vi "tasklist_wait.vi"(8 "error in (no error)":errorcluster, 11 "pid":i32) -> (0 "error out":errorcluster)   [LabVIEW 2015, in "lv-bin-windows.lvlib" / "v1.lvlib"]
uses:
  v1.lvlib
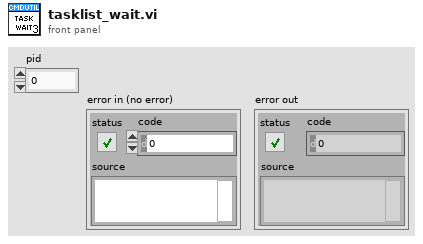
[diagram p1: front panel]
types:
  T1 = cluster{"image_name []":string[], "pid []":i32[], "session_name []":string[], "session_number []":i32[], "memory_usage []":dbl[]}
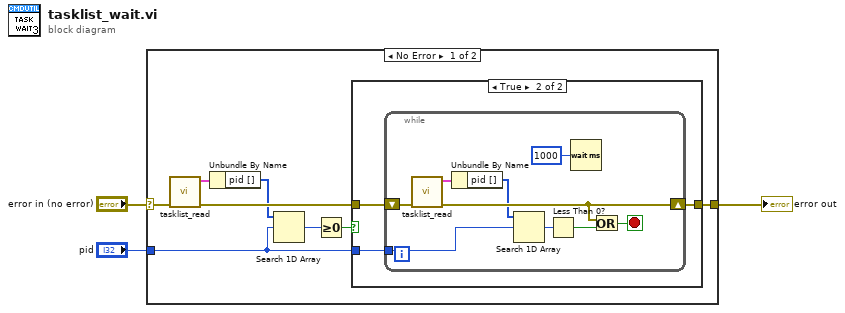
[diagram p0: block diagram]
diagram:
  n1 = case shown="No Error" "error in (no error)" {
    selector: "error in (no error)" -> [w6 w25]
    tunnel: "pid" -> [w7 _]
    tunnel: [w5 w25] -> w1
    frame No Error {
      n2 = call "tasklist_read.vi"("error in (no error)"=w6) -> ("error out"=w11:errorcluster, "tasklist"=w10:T1)  [unwired: 9 in]
      n3 = Unbundle By Name(w10) -> ("pid []"=w9:i32[])
      n4 = Search 1D Array(1D array=w9, element=w7) -> (index of element=w8:i32)  [unwired: 1 in]
      n5 = Greater Or Equal To 0?(x=w8) -> (x >= 0?=w4:bool)
      n6 = case shown="True" w4 {
        tunnel: w11 -> [w12 w15]
        tunnel: w7 -> [_ w14]
        tunnel: [w12 w13] -> w5
        frame False {
        }
        frame True {
          n7 = while {
            tunnel: w14 -> [w16]
            shift-right: [w24] -> w13
            shift-left: w15 -> [w17]
            stop <- w18 stop-if-true
            n8 = call "tasklist_read.vi"("error in (no error)"=w17) -> ("error out"=w24:errorcluster, "tasklist"=w21:T1)  [unwired: 9 in]
            n9 = Unbundle By Name(w21) -> ("pid []"=w22:i32[])
            n10 = Search 1D Array(1D array=w22, element=w16) -> (index of element=w23:i32)  [unwired: 1 in]
            n11 = Less Than 0?(x=w23) -> (x < 0?=w19:bool)
            n12 = Wait (ms)(milliseconds to wait=u32 1000) -> ()  [unwired: 1 out]
            n13 = Or(x=w24, y=w19) -> (x .or. y?=w18:bool)
          }
        }
      }
    }
    frame Error {
    }
  }
  "error out" <- w1
